vi "Numeros aleatorios.vi"() -> ()   [LabVIEW 2024]
panel:
  out "number (0 to 1)":dbl
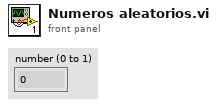
[diagram p1: front panel]
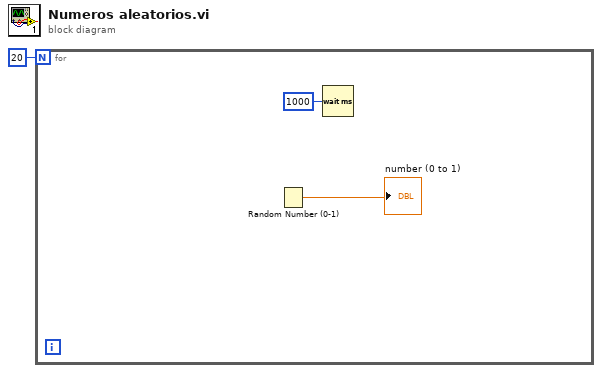
[diagram p0: block diagram]
diagram:
  n1 = for {
    N: 20 -> [_]
    n2 = Random Number (0-1)() -> (number: 0 to 1=→"number (0 to 1)":dbl)
    n3 = Wait (ms)(milliseconds to wait=u32 1000) -> ()  [unwired: 1 out]
  }
